vi "Amplitude Spectrum PtbyPt.vi"() -> ()   [LabVIEW 2023]
doc: "This VI shows the difference in action between point-by-point and block-oriented amplitude spectrums by running the two side by side. The input data is simulated by two sine waves plus Gaussian noise."
uses:
  <vilib>/ptbypt/NI_PtbyPt.lvlib
  <vilib>/Analysis/NI_AALPro.lvlib
panel:
  in  "Frequency 2":dbl(slide)=0.34563758389261745 scale=0.0..0.5 scale format="%0.1f"
  out "Acquired block":bool
  out "Block-Oriented Amplitude Spectrum":T1(graph)
  out "Point-by-Point Amplitude Spectrum":T1(graph)
  in  "Noise level":dbl(slide)=0.9054054054054055 scale=0.0..2.0 scale format="%#.2f"
  in  "Frequency 1":dbl(slide)=0.17757009345794392 scale=0.0..0.5 scale format="%0.1f"
  in  "Block Length":i32=500 min=1
  in  "Stop":bool
  # "Overview: This VI shows the difference in action between point-by-point and block-oriented amplitude spectrum by running the two side by side.\nRequirement: LabVIEW Full Development System\nInstructions: \n1. Run the VI.\n2. Change parameters of the input signals ( Frequency 1, Frequency 2 and Noise level). Notice that the Point-by-Point Amplitude Spectrum graph updates with every new sample, and the Block-oriented Amplitude Spectrum graph will only update after the number of samples in the Block length has been reached.\n3. Click Stop to stop the VI."
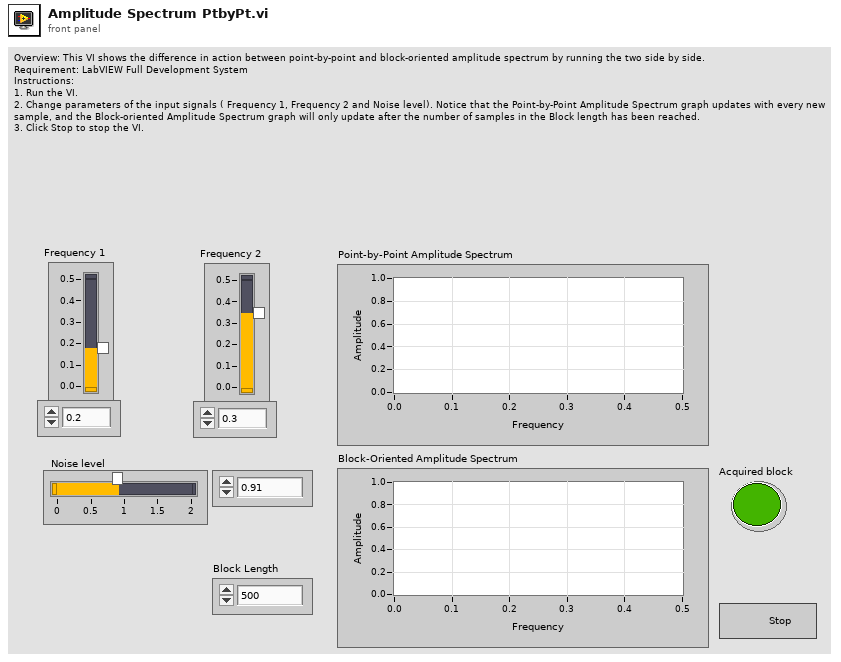
[diagram p1: front panel]
types:
  T1 = cluster{dbl, "df":dbl, "Amp Spectrum Mag (Vrms)":dbl[]}
  T2 = cluster{"df":dbl, "df":dbl, "Amp Spectrum Mag (Vrms)":dbl[]}
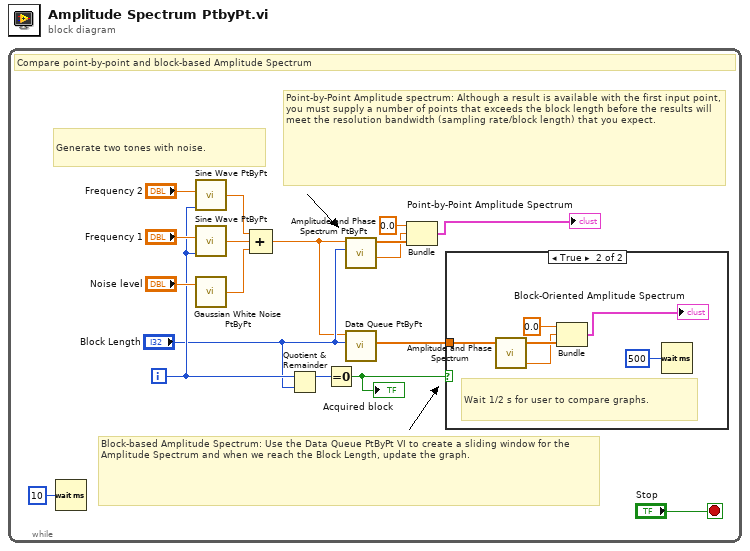
[diagram p0: block diagram]
diagram:
  n1 = while {
    i -> [w10]
    stop <- "Stop" stop-if-true
    # "Block-based Amplitude Spectrum: Use the Data Queue PtByPt VI to create a sliding window for the Amplitude Spectrum and when we reach the Block Length, update the graph."
    # "Generate two tones with noise."
    # "Point-by-Point Amplitude spectrum: Although a result is available with the first input point, you must supply a number of points that exceeds the block length before the results will meet the resolution bandwidth (sampling rate/block length) that you expect."
    # "Compare point-by-point and block-based Amplitude Spectrum"
    n2 = Wait (ms)(milliseconds to wait=u32 10) -> ()  [unwired: 1 out]
    n3 = call <vilib>:"Sine Wave PtByPt.vi"("time"=w10, "frequency"="Frequency 2") -> ("sine wave"=w5:dbl)  [unwired: 2 in]
    n4 = call <vilib>:"Sine Wave PtByPt.vi"("time"=w10, "frequency"="Frequency 1") -> ("sine wave"=w4:dbl)  [unwired: 2 in]
    n5 = call <vilib>:"Gaussian White Noise PtByPt.vi"("standard deviation"="Noise level") -> ("Gaussian white noise"=w3:dbl)  [unwired: 2 in]
    n6 = Compound Arithmetic op=ADD(w5, w4, w3) -> (w2:dbl)
    n7 = Quotient & Remainder(x=w10, y="Block Length") -> (x-y*floor(x/y)=w8:i32)  [unwired: 1 out]
    n8 = Equal To 0?(x=w8) -> (x = 0?=w7:bool)
    "Acquired block" <- w7
    n9 = call <vilib>:"Amplitude and Phase Spectrum PtByPt.vi"("sample length"="Block Length", "signal"=w2) -> ("df"=w15:dbl, "Amp Spectrum Mag (Vrms)"=w16:dbl[])  [unwired: 3 in, 2 out]
    n10 = call <vilib>:"Data Queue PtByPt.vi"("sample length"="Block Length", "input data point"=w2) -> ("Current Queue"=w11:dbl[])  [unwired: 5 in, 4 out]
    n11 = Bundle("df"=0.0, "df"=w15, "Amp Spectrum Mag (Vrms)"=w16) -> (→"Point-by-Point Amplitude Spectrum":T2)  [unwired: 1 in]
    n12 = case shown="True" w7 {
      tunnel: w11 -> [_ w22]
      frame False {
      }
      frame True {
        # "Wait 1/2 s for user to compare graphs."
        n13 = call <vilib>:"Amplitude and Phase Spectrum.vi"("Signal (V)"=w22) -> ("df"=w23:dbl, "Amp Spectrum Mag (Vrms)"=w24:dbl[])  [unwired: 2 in, 1 out]
        n14 = Bundle("df"=0.0, "df"=w23, "Amp Spectrum Mag (Vrms)"=w24) -> (→"Block-Oriented Amplitude Spectrum":T2)  [unwired: 1 in]
        n15 = Wait (ms)(milliseconds to wait=u32 500) -> ()  [unwired: 1 out]
      }
    }
  }
